vi "time_to_match_activity_15.vi"() -> ()   [LabVIEW 2025]
panel:
  out "Time to Match":dbl format="%#.3g"
  out "# of iterations":i32
  out "Current Number":i32
  in  "Number to Match":i32 min=0 max=100 step=1
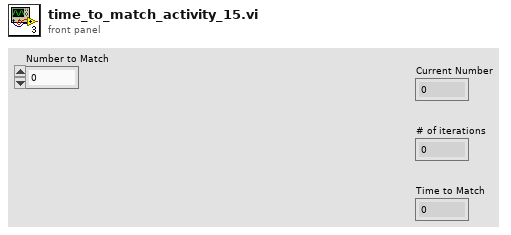
[diagram p1: front panel]
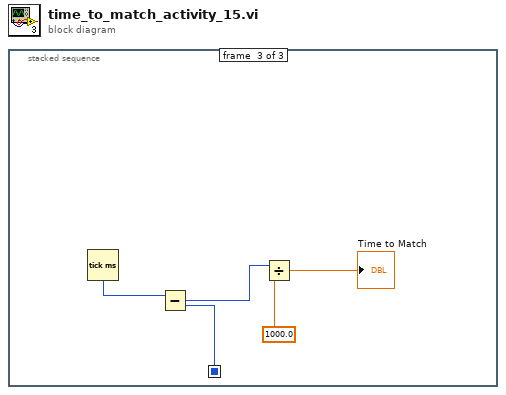
[diagram p0: block diagram]
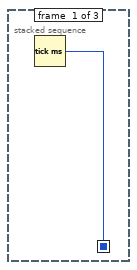
[diagram p2: hidden frame]
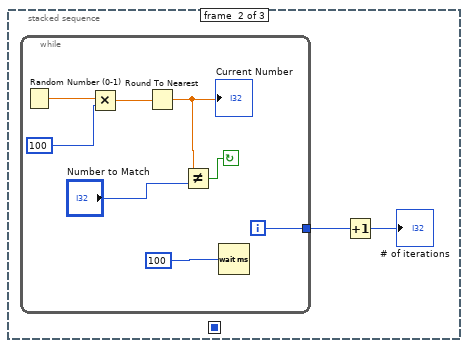
[diagram p3: hidden frame]
diagram:
  n1 = stacked-sequence {
    seq-local: [w1 _ _] -> [_ _ w13]
    frame #0 {
      n2 = Tick Count (ms)() -> (millisecond timer value=w1:u32)
    }
    frame #1 {
      n3 = while {
        tunnel: [w5] -> w2
        i -> [w5]
        stop <- w8 continue-if-true
        n4 = Random Number (0-1)() -> (number: 0 to 1=w11:dbl)
        n5 = Multiply(x=w11, y=100) -> (x*y=w7:dbl)
        n6 = Round To Nearest(number=w7) -> (nearest integer value=w6:dbl)
        "Current Number" <- w6
        n7 = Not Equal?(x=w6, y="Number to Match") -> (x != y?=w8:bool)
        n8 = Wait (ms)(milliseconds to wait=100) -> ()  [unwired: 1 out]
      }
      n9 = Increment(x=w2) -> (x+1=→"# of iterations":i32)
    }
    frame #2 {
      n10 = Tick Count (ms)() -> (millisecond timer value=w16:u32)
      n11 = Subtract(x=w16, y=w13) -> (x-y=w15:u32)
      n12 = Divide(x=w15, y=1000.0) -> (x/y=→"Time to Match":dbl)
    }
  }
